vi "GenesysPS.ProcCases.vi"(0 "i ref in":refnum<vi>, 1 "selector":string, 2 "Data":T1, 3 "call cluster":T2={"Object"="", "Selector"="", "CallType"=enum."synchronous", "Async Object"="", "Async Selector"="", "Data Descriptor"="", "Data"=[], "Error #"=0, "Expire"=0}, 5 "error in (no error)":errorcluster) -> (14 "i ref out":refnum<vi>, 17 "answer cluster":T2={"Object"="", "Selector"="", "CallType"=enum."synchronous", "Async Object"="", "Async Selector"="", "Data Descriptor"="", "Data"=[], "Error #"=0, "Expire"=0}, 19 "error out":errorcluster)   [LabVIEW 2014, in "GenesysPS.lvlib"]
doc: "This method is called by a process from within the default case in the event loop. The methods of a class that are linked to events will be called from THIS method. Add your code here."
uses:
  GenesysPS.lvlib
  CSCore/CSSystem/CoreLib/CoreLib.lvlib
  CSCore/BaseProcess/BaseProcess.lvlib
  DIMPowerSupply/DIMPowerSupply.lvlib
  CSCore/CSSystem/CoreLib/CoreLib.string 2 byte array.vi
  CSCore/CSSystem/CoreLib/CoreLib.byte array 2 short.vi
  CSCore/CSSystem/CoreLib/CoreLib.double 2 byte array.vi
  CSCore/CSApplicationBaseClasses/PSChannelBase/PSChannelBase.lvlib
  CSCore/CSSystem/CoreDefs/CoreDefs.call_type.ctl
  CSCore/CSSystem/CoreDefs/CoreDefs.rawDataType.ctl
  CSCore/BaseProcess/BaseProcess.descriptor string definition.ctl
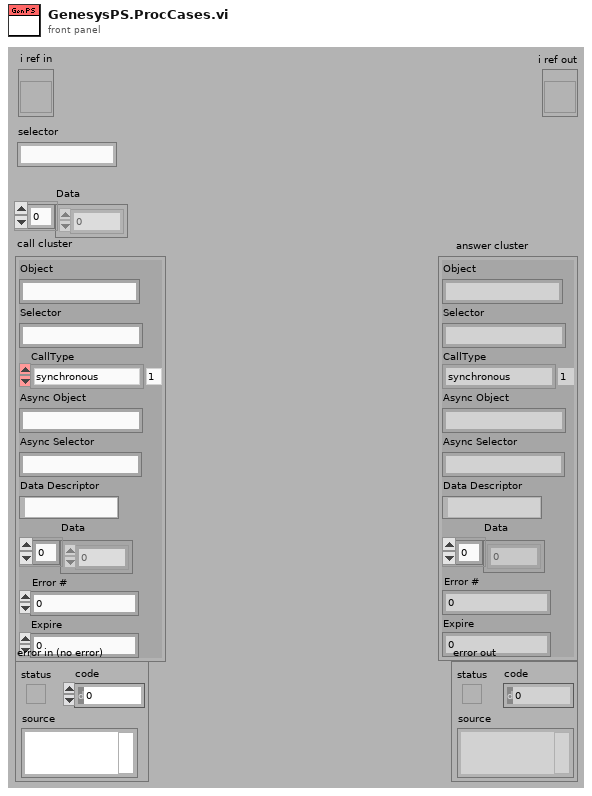
[diagram p1: front panel]
types:
  T1 = typedef "CoreDefs.rawDataType.ctl" = i8[]
  T2 = typedef "CoreDefs.call_type.ctl" = cluster{"Object":string, "Selector":string, "CallType":enum16{"simple", "synchronous", "asynchronous"}, "Async Object":string, "Async Selector":string, "Data Descriptor":T3, "Data":T1, "Error #":i32, "Expire":u32}
  T3 = typedef "BaseProcess.lvlib/BaseProcess.descriptor string definition.ctl" = string
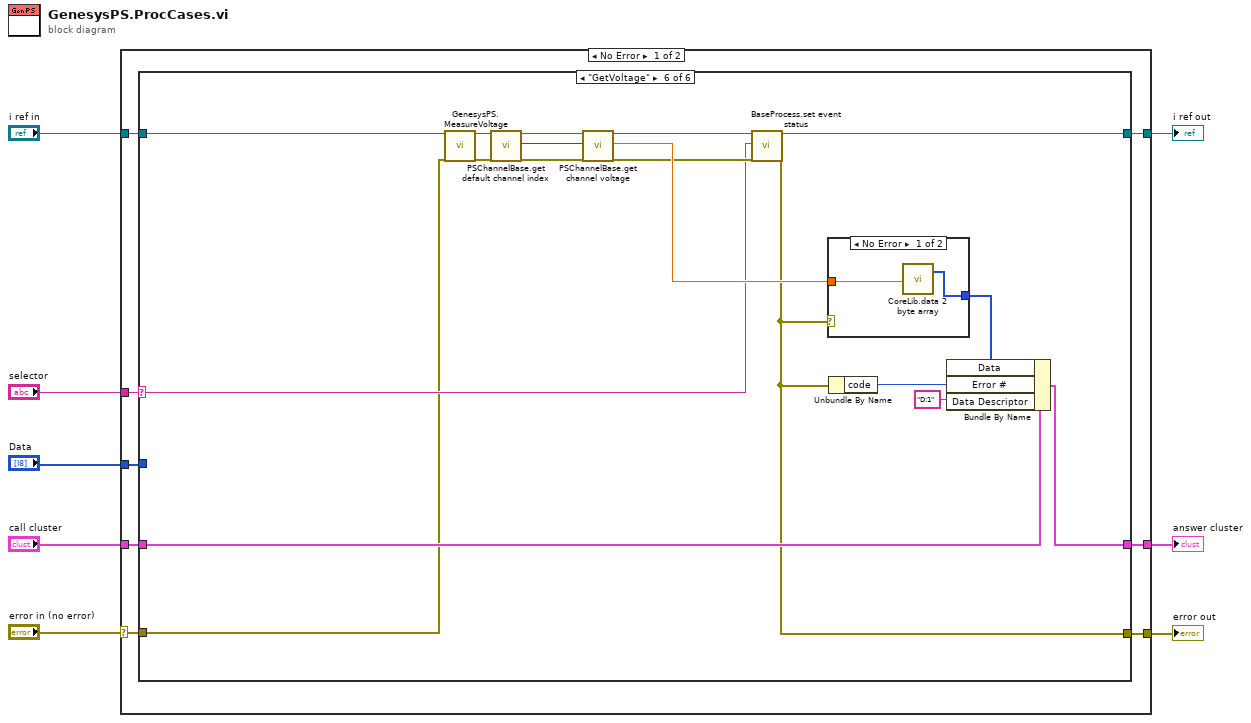
[diagram p0: block diagram]
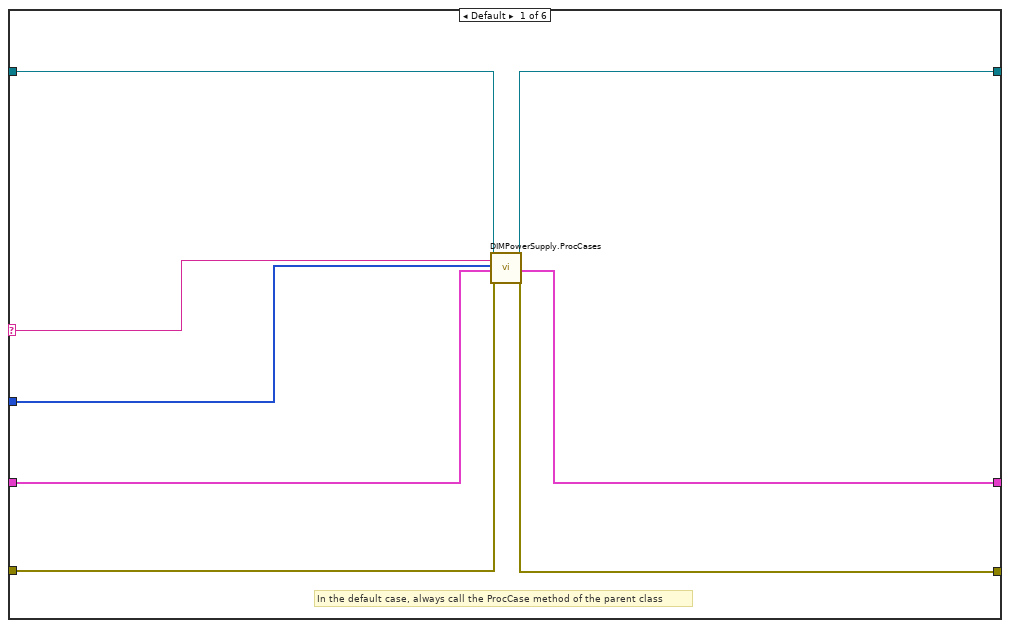
[diagram p2: hidden frame]
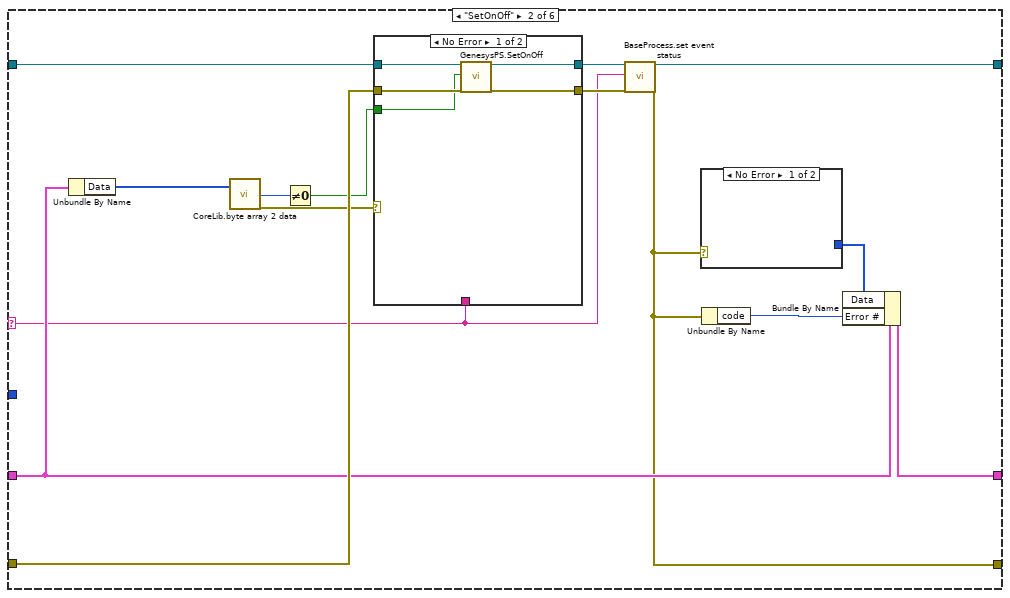
[diagram p3: hidden frame]
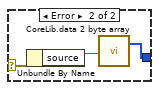
[diagram p4: hidden frame]
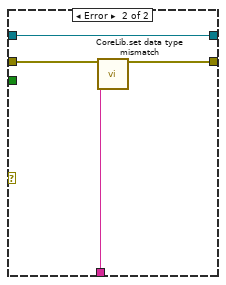
[diagram p5: hidden frame]
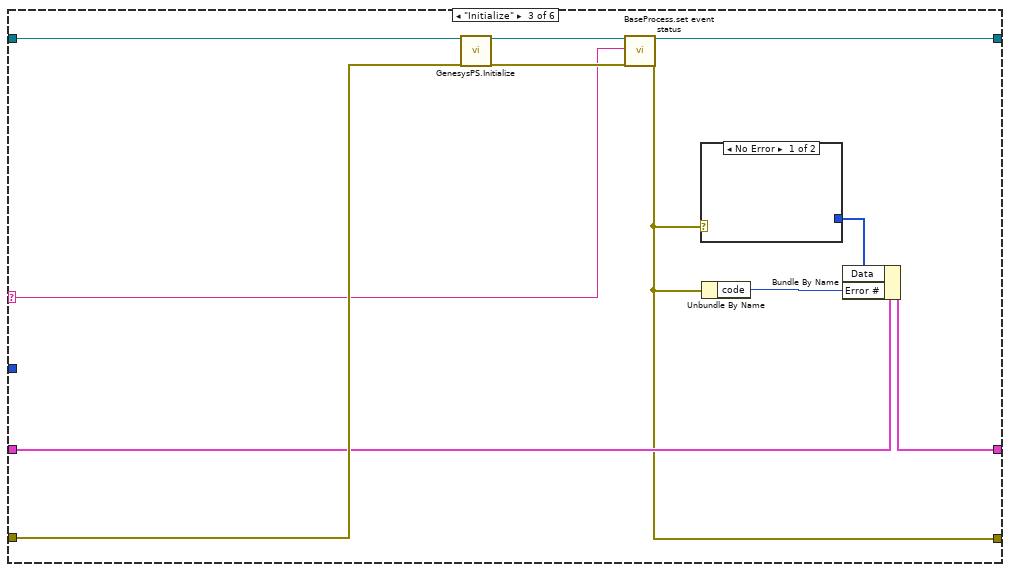
[diagram p6: hidden frame]
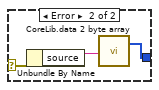
[diagram p7: hidden frame]
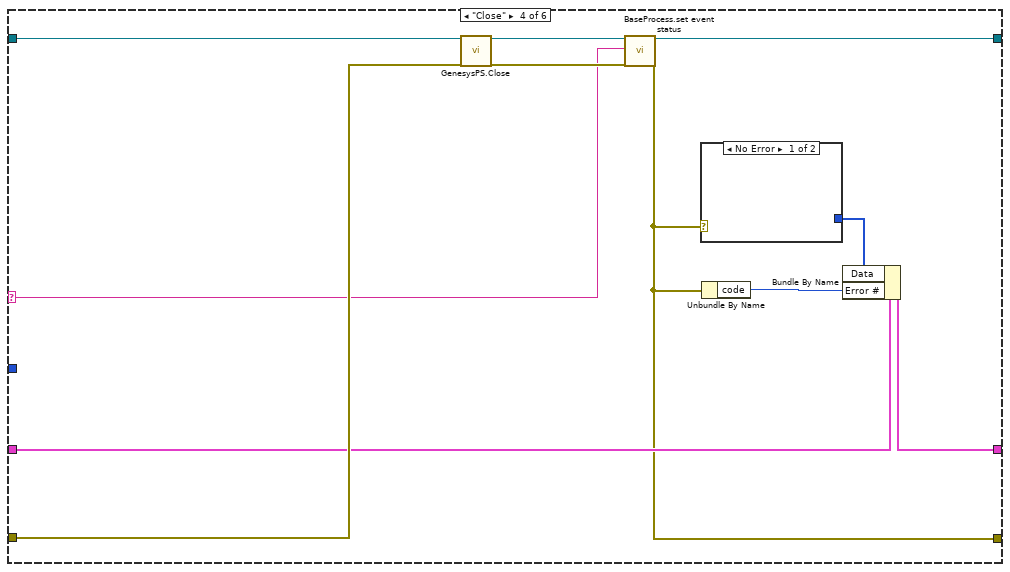
[diagram p8: hidden frame]
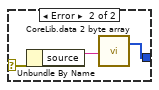
[diagram p9: hidden frame]
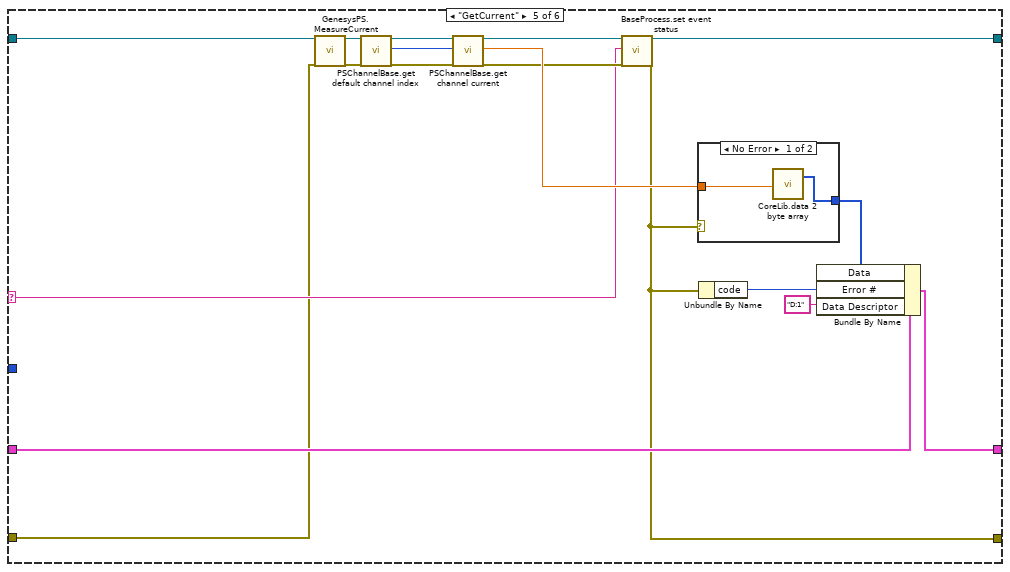
[diagram p10: hidden frame]
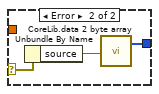
[diagram p11: hidden frame]
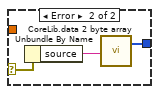
[diagram p12: hidden frame]
diagram:
  n1 = case shown="No Error" "error in (no error)" {
    selector: "error in (no error)" -> [w9 w126]
    tunnel: "selector" -> [w16 _]
    tunnel: [w15 w127] -> w7
    tunnel: "Data" -> [w14 _]
    tunnel: "call cluster" -> [w13 w127]
    tunnel: "i ref in" -> [w12 w128]
    tunnel: [w11 w128] -> w3
    tunnel: [w10 w126] -> w2
    frame No Error {
      n2 = case shown="\"GetVoltage\"" w16 {
        selector: w16 -> [w18 w30 w53 w67 w85 w108]
        tunnel: w14 -> [w19 _ _ _ _ _]
        tunnel: w12 -> [w17 w39 w62 w76 w82 w105]
        tunnel: [w24 w29 w52 w66 w84 w107] -> w11
        tunnel: w13 -> [w20 w36 w59 w73 w88 w111]
        tunnel: [w21 w35 w58 w72 w87 w110] -> w15
        tunnel: w9 -> [w23 w38 w61 w75 w81 w104]
        tunnel: [w22 w31 w54 w68 w86 w109] -> w10
        frame Default {
          # "In the default case, always call the ProcCase method of the parent class"
          n3 = call "DIMPowerSupply.ProcCases.vi"("i ref in"=w17, "selector"=w18, "Data"=w19, "call cluster"=w20, "error in (no error)"=w23) -> ("i ref out"=w24:refnum<vi>, "answer cluster"=w21:T2, "error out"=w22:errorcluster)  [unwired: 12 in]
        }
        frame "SetOnOff" {
          n4 = Unbundle By Name(w36) -> ("Data"=w27:T1)
          n5 = call-poly "CoreLib.byte array 2 data.vi"("byteArray"=w27) -> ("i16"=w26:i16, "error out"=w28:errorcluster)  [unwired: 16 in, 1 out]
          n6 = Not Equal To 0?(x=w26) -> (x != 0?=w25:bool)
          n7 = case shown="No Error" w28 {
            tunnel: [w45 w51] -> w33
            tunnel: w39 -> [w44 w51]
            tunnel: w38 -> [w47 w50]
            tunnel: [w46 w49] -> w32
            tunnel: w30 -> [_ w48]
            tunnel: w25 -> [w43 _]
            frame No Error {
              n8 = call "GenesysPS.SetOnOff.vi"("i ref in"=w44, "on (FALSE)"=w43, "error in (no error)"=w47) -> ("i ref out"=w45:refnum<vi>, "error out"=w46:errorcluster)  [unwired: 15 in]
            }
            frame Error {
              n9 = call "CoreLib.set data type mismatch.vi"("error in (no error)"=w50, "error source"=w48) -> ("error out"=w49:errorcluster)  [unwired: 17 in]
            }
          }
          n10 = call "BaseProcess.set event status.vi"("i ref in"=w33, "EventStatus"=w30, "error in (no error)"=w32) -> ("i ref out"=w29:refnum<vi>, "error out"=w31:errorcluster)  [unwired: 14 in, 1 out]
          n11 = case shown="No Error" w31 {
            selector: w31 -> [_ w42]
            tunnel: [_ w40] -> w34
            frame No Error {
            }
            frame Error {
              n12 = Unbundle By Name(w42) -> ("source"=w41:string)
              n13 = call-poly "CoreLib.data 2 byte array.vi"("string"=w41) -> ("byteArray out"=w40:T1)  [unwired: 18 in]
            }
          }
          n14 = Unbundle By Name(w31) -> ("code"=w37:i32)
          n15 = Bundle By Name(cluster=w36, "Data"=w34, "Error #"=w37) -> (w35:T2)
        }
        frame "Initialize" {
          n16 = call "GenesysPS.Initialize.vi"("i ref in"=w62, "error in (no error)"=w61) -> ("i ref out"=w56:refnum<vi>, "error out"=w55:errorcluster)  [unwired: 16 in]
          n17 = call "BaseProcess.set event status.vi"("i ref in"=w56, "EventStatus"=w53, "error in (no error)"=w55) -> ("i ref out"=w52:refnum<vi>, "error out"=w54:errorcluster)  [unwired: 14 in, 1 out]
          n18 = case shown="No Error" w54 {
            selector: w54 -> [_ w65]
            tunnel: [_ w63] -> w57
            frame No Error {
            }
            frame Error {
              n19 = Unbundle By Name(w65) -> ("source"=w64:string)
              n20 = call-poly "CoreLib.data 2 byte array.vi"("string"=w64) -> ("byteArray out"=w63:T1)  [unwired: 18 in]
            }
          }
          n21 = Unbundle By Name(w54) -> ("code"=w60:i32)
          n22 = Bundle By Name(cluster=w59, "Data"=w57, "Error #"=w60) -> (w58:T2)
        }
        frame "Close" {
          n23 = call "GenesysPS.Close.vi"("i ref in"=w76, "error in (no error)"=w75) -> ("i ref out"=w70:refnum<vi>, "error out"=w69:errorcluster)  [unwired: 16 in]
          n24 = call "BaseProcess.set event status.vi"("i ref in"=w70, "EventStatus"=w67, "error in (no error)"=w69) -> ("i ref out"=w66:refnum<vi>, "error out"=w68:errorcluster)  [unwired: 14 in, 1 out]
          n25 = case shown="No Error" w68 {
            selector: w68 -> [_ w79]
            tunnel: [_ w77] -> w71
            frame No Error {
            }
            frame Error {
              n26 = Unbundle By Name(w79) -> ("source"=w78:string)
              n27 = call-poly "CoreLib.data 2 byte array.vi"("string"=w78) -> ("byteArray out"=w77:T1)  [unwired: 18 in]
            }
          }
          n28 = Unbundle By Name(w68) -> ("code"=w74:i32)
          n29 = Bundle By Name(cluster=w73, "Data"=w71, "Error #"=w74) -> (w72:T2)
        }
        frame "GetCurrent" {
          n30 = call "GenesysPS.MeasureCurrent.vi"("i ref in"=w82, "error in (no error)"=w81) -> ("i ref out"=w83:refnum<vi>, "error out"=w80:errorcluster)  [unwired: 16 in]
          n31 = call "PSChannelBase.get default channel index.vi"("i ref in"=w83, "error in (no error)"=w80) -> ("i ref out"=w89:refnum<vi>, "defaultChannelIndex"=w90:i32, "error out"=w91:errorcluster)  [unwired: 15 in]
          n32 = call "PSChannelBase.get channel current.vi"("i ref in"=w89, "channelIndx"=w90, "error in (no error)"=w91) -> ("i ref out"=w94:refnum<vi>, "current"=w97:dbl, "error out"=w93:errorcluster)  [unwired: 14 in]
          n33 = call "BaseProcess.set event status.vi"("i ref in"=w94, "EventStatus"=w85, "error in (no error)"=w93) -> ("i ref out"=w84:refnum<vi>, "error out"=w86:errorcluster)  [unwired: 14 in, 1 out]
          n34 = case shown="No Error" w86 {
            selector: w86 -> [_ w102]
            tunnel: [w99 w101] -> w95
            tunnel: w97 -> [w98 _]
            frame No Error {
              n35 = call-poly "CoreLib.data 2 byte array.vi"("f64"=w98) -> ("byteArray out"=w99:T1)  [unwired: 18 in]
            }
            frame Error {
              n36 = Unbundle By Name(w102) -> ("source"=w100:string)
              n37 = call-poly "CoreLib.data 2 byte array.vi"("string"=w100) -> ("byteArray out"=w101:T1)  [unwired: 18 in]
            }
          }
          n38 = Unbundle By Name(w86) -> ("code"=w96:i32)
          n39 = Bundle By Name(cluster=w88, "Data"=w95, "Error #"=w96, "Data Descriptor"="D:1") -> (w87:T2)
        }
        frame "GetVoltage" {
          n40 = call "GenesysPS.MeasureVoltage.vi"("i ref in"=w105, "error in (no error)"=w104) -> ("i ref out"=w106:refnum<vi>, "error out"=w103:errorcluster)  [unwired: 16 in]
          n41 = call "PSChannelBase.get default channel index.vi"("i ref in"=w106, "error in (no error)"=w103) -> ("i ref out"=w112:refnum<vi>, "defaultChannelIndex"=w113:i32, "error out"=w114:errorcluster)  [unwired: 15 in]
          n42 = call "PSChannelBase.get channel voltage.vi"("i ref in"=w112, "channelIndx"=w113, "error in (no error)"=w114) -> ("i ref out"=w117:refnum<vi>, "voltage"=w120:dbl, "error out"=w116:errorcluster)  [unwired: 14 in]
          n43 = call "BaseProcess.set event status.vi"("i ref in"=w117, "EventStatus"=w108, "error in (no error)"=w116) -> ("i ref out"=w107:refnum<vi>, "error out"=w109:errorcluster)  [unwired: 14 in, 1 out]
          n44 = case shown="No Error" w109 {
            selector: w109 -> [_ w125]
            tunnel: [w122 w124] -> w118
            tunnel: w120 -> [w121 _]
            frame No Error {
              n45 = call-poly "CoreLib.data 2 byte array.vi"("f64"=w121) -> ("byteArray out"=w122:T1)  [unwired: 18 in]
            }
            frame Error {
              n46 = Unbundle By Name(w125) -> ("source"=w123:string)
              n47 = call-poly "CoreLib.data 2 byte array.vi"("string"=w123) -> ("byteArray out"=w124:T1)  [unwired: 18 in]
            }
          }
          n48 = Unbundle By Name(w109) -> ("code"=w119:i32)
          n49 = Bundle By Name(cluster=w111, "Data"=w118, "Error #"=w119, "Data Descriptor"="D:1") -> (w110:T2)
        }
      }
    }
    frame Error {
    }
  }
  "answer cluster" <- w7
  "i ref out" <- w3
  "error out" <- w2
